vi "VIP_Pre-Install Custom Action.vi"(10 "Variant":variant) -> (0 "error out":errorcluster)   [LabVIEW 2021]
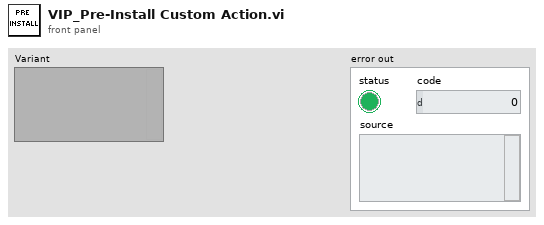
[diagram p1: front panel]
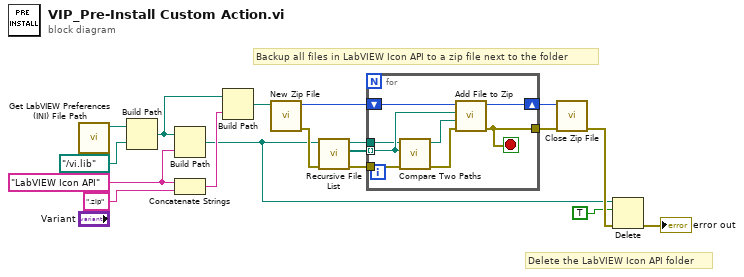
[diagram p0: block diagram]
diagram:
  w6 = "LabVIEW Icon API"
  # "Delete the LabVIEW Icon API folder"
  # "Backup all files in LabVIEW Icon API to a zip file next to the folder"
  n1 = call <resource>:"Get LabVIEW Preferences (INI) File Path.vi"() -> ("LabVIEW Preferences (INI) File Path"=w8:path)  [unwired: 11 in]
  n2 = Build Path(base path=w8, name or relative path=path "../vi.lib" ("symbolic path")) -> (appended path=w4:path)
  n3 = Build Path(base path=w4, name or relative path=w6) -> (appended path=w1:path)
  n4 = Concatenate Strings(w6, ".zip" ("string")) -> (w3:string)
  n5 = Build Path(base path=w4, name or relative path=w3) -> (appended path=w2:path)
  n6 = call <vilib>:"New Zip File.vi"("target"=w2) -> ("error out"=w15:errorcluster, "zip file out"=w11:i64)  [unwired: 4 in, 1 out]
  n7 = call <vilib>:"Recursive File List.vi"("error in (no error)"=w15, "Folder Path"=w1) -> ("error out"=w16:errorcluster, "All Files in Dir"=w13:path[], "dup Folder Path"=w9:path)  [unwired: 5 in, 2 out]
  n8 = for {
    tunnel: w13 -> [w21] mode=indexing
    tunnel: w16 -> [w25]
    tunnel: [w26] -> w17
    shift-right: [w22] -> w12
    shift-left: w11 -> [w23]
    tunnel: w9 -> [w20]
    stop <- w26 stop-if-true
    n9 = call <vilib>:"Compare Two Paths.vi"("error in (no error)"=w25, "Path 2"=w21, "Path 1"=w20) -> ("error out"=w24:errorcluster, "Relative Path from 1 to 2"=w19:path)  [unwired: 5 in, 2 out]
    n10 = call <vilib>:"Add File to Zip.vi"("error in (no error)"=w24, "destination path in zip"=w19, "source file path"=w21, "zip file in"=w23) -> ("error out"=w26:errorcluster, "zip file out"=w22:i64)  [unwired: 6 out]
  }
  n11 = call <vilib>:"Close Zip File.vi"("error in (no error)"=w17, "zip file in"=w12) -> ("error out"=w18:errorcluster)  [unwired: 5 in]
  n12 = Delete(path (use dialog)=w1, entire hierarchy (F)=TRUE, error in=w18) -> (error out=→"error out":errorcluster)  [unwired: 2 in, 2 out]
